vi "AuMT8852B EDR Carrier Frequency and Modulation Configuration.vi"(5 "Settings":T1={"Low frequency selection"=enum."Use low frequency", "Medium frequency selection"=enum."Use medium frequency", "High frequency selection"=enum."Use high frequency", "Low TX frequency"=2402.0, "Low RX frequency"=2480.0, "Medium TX frequency"=2441.0, "Medium RX frequency"=2402.0, "High TX frequency"=2480.0, "High RX frequency"=2402.0, "Number of blocks"=200, "Initial frequency error lower limit"=-75000.0, "Initial frequency error upper limit"=75000.0, "2DHx test packet"=enum."Longest", "3DHx test packet"=enum."Longest", "Hop selection"=enum."Test with hopping off", "Test control"=enum."Loopback", "Hop mode"=enum."Defined", "Frequency error lower limit"=-10000.0, "Frequency error upper limit"=10000.0, "Block frequency error lower limit"=-75000.0, "Block frequency error upper limit"=75000.0, "2Mbs RMS DEVM limit"=0.2, "3Mbs RMS DEVM limit"=0.13, "2Mbs peak DEVM limit"=0.35000000000000014, "3Mbs peak DEVM limit"=0.25, "2Mbs 99% packets DEVM limit"=0.3, "3Mbs 99% packets DEVM limit"=0.2} {"3Mbs 99% packets DEVM limit" min=0.0 max=1.0 step=0.01 format="%.2f"; "2Mbs 99% packets DEVM limit" min=0.0 max=1.0 step=0.01 format="%.2f"; "3Mbs peak DEVM limit" min=0.0 max=1.0 step=0.01 format="%.2f"; "2Mbs peak DEVM limit" min=0.0 max=1.0 step=0.01 format="%.2f"; "3Mbs RMS DEVM limit" min=0.0 max=1.0 step=0.01 format="%.2f"; "2Mbs RMS DEVM limit" min=0.0 max=1.0 step=0.01 format="%.2f"; "Block frequency error upper limit" min=-100000.0 max=100000.0 step=1000.0 format="%#.0f"; "Block frequency error lower limit" min=-100000.0 max=100000.0 step=1000.0 format="%#.2f"; "Frequency error upper limit" min=-100000.0 max=100000.0 step=1000.0 format="%#.0f"; "Frequency error lower limit" min=-100000.0 max=100000.0 step=1000.0 format="%#.0f"; "Initial frequency error upper limit" min=-100000.0 max=100000.0 step=1000.0 format="%#.0f"; "Initial frequency error lower limit" min=-100000.0 max=100000.0 step=1000.0 format="%#.0f"}, 7 "Set/Get (Set)":enum16{"Set", "Get"}(ring), 8 "error in (no error)":errorcluster, 10 "Script (3)":i32=3, 11 "VISA session":refnum<visa-resource-name>) -> (0 "error out":errorcluster, 2 "error code":i32, 3 "VISA session out":refnum<visa-resource-name>, 4 "Settings out":T1={"Low frequency selection"=enum."Use low frequency", "Medium frequency selection"=enum."Use medium frequency", "High frequency selection"=enum."Use high frequency", "Low TX frequency"=2402.0, "Low RX frequency"=2480.0, "Medium TX frequency"=2441.0, "Medium RX frequency"=2402.0, "High TX frequency"=2480.0, "High RX frequency"=2402.0, "Number of blocks"=200, "Initial frequency error lower limit"=-75000.0, "Initial frequency error upper limit"=75000.0, "2DHx test packet"=enum."Longest", "3DHx test packet"=enum."Longest", "Hop selection"=enum."Test with hopping off", "Test control"=enum."Loopback", "Hop mode"=enum."Defined", "Frequency error lower limit"=-10000.0, "Frequency error upper limit"=10000.0, "Block frequency error lower limit"=-75000.0, "Block frequency error upper limit"=75000.0, "2Mbs RMS DEVM limit"=0.2, "3Mbs RMS DEVM limit"=0.13, "2Mbs peak DEVM limit"=0.35000000000000014, "3Mbs peak DEVM limit"=0.25, "2Mbs 99% packets DEVM limit"=0.3, "3Mbs 99% packets DEVM limit"=0.2} {"3Mbs 99% packets DEVM limit" format="%.2f"; "2Mbs 99% packets DEVM limit" format="%.2f"; "3Mbs peak DEVM limit" format="%.2f"; "2Mbs peak DEVM limit" format="%.2f"; "3Mbs RMS DEVM limit" format="%.2f"; "2Mbs RMS DEVM limit" format="%.2f"; "Block frequency error upper limit" format="%#.2f"; "Block frequency error lower limit" format="%#.2f"; "Frequency error upper limit" format="%#.2f"; "Frequency error lower limit" format="%#.2f"; "Initial frequency error upper limit" format="%#.0f"; "Initial frequency error lower limit" format="%#.2f"})   [LabVIEW 2017]
doc: "Anritsu MT8852B Bluetooth Tester\n\nConfigures the instrument for the EDR Carrier Frequency Stability and Modulation test.\n\nINPUTS\nSet/Get - whether the values are being sent to or retrieved from the instrument.\nScript - which of the stored scripts (1-10) will be queried or configured. Scripts 1 and 2 are read-only.\nSettings - parameters of the test to be written.\n\nOUTPUTS\nSettings out - current parameters of the test."
uses:
  <instrlib>/aumt8852B/General/Utilities/MT8850 Test Parameters.ctl
  <instrlib>/aumt8852B/General/Utilities/MT8850 Frequency Units.ctl
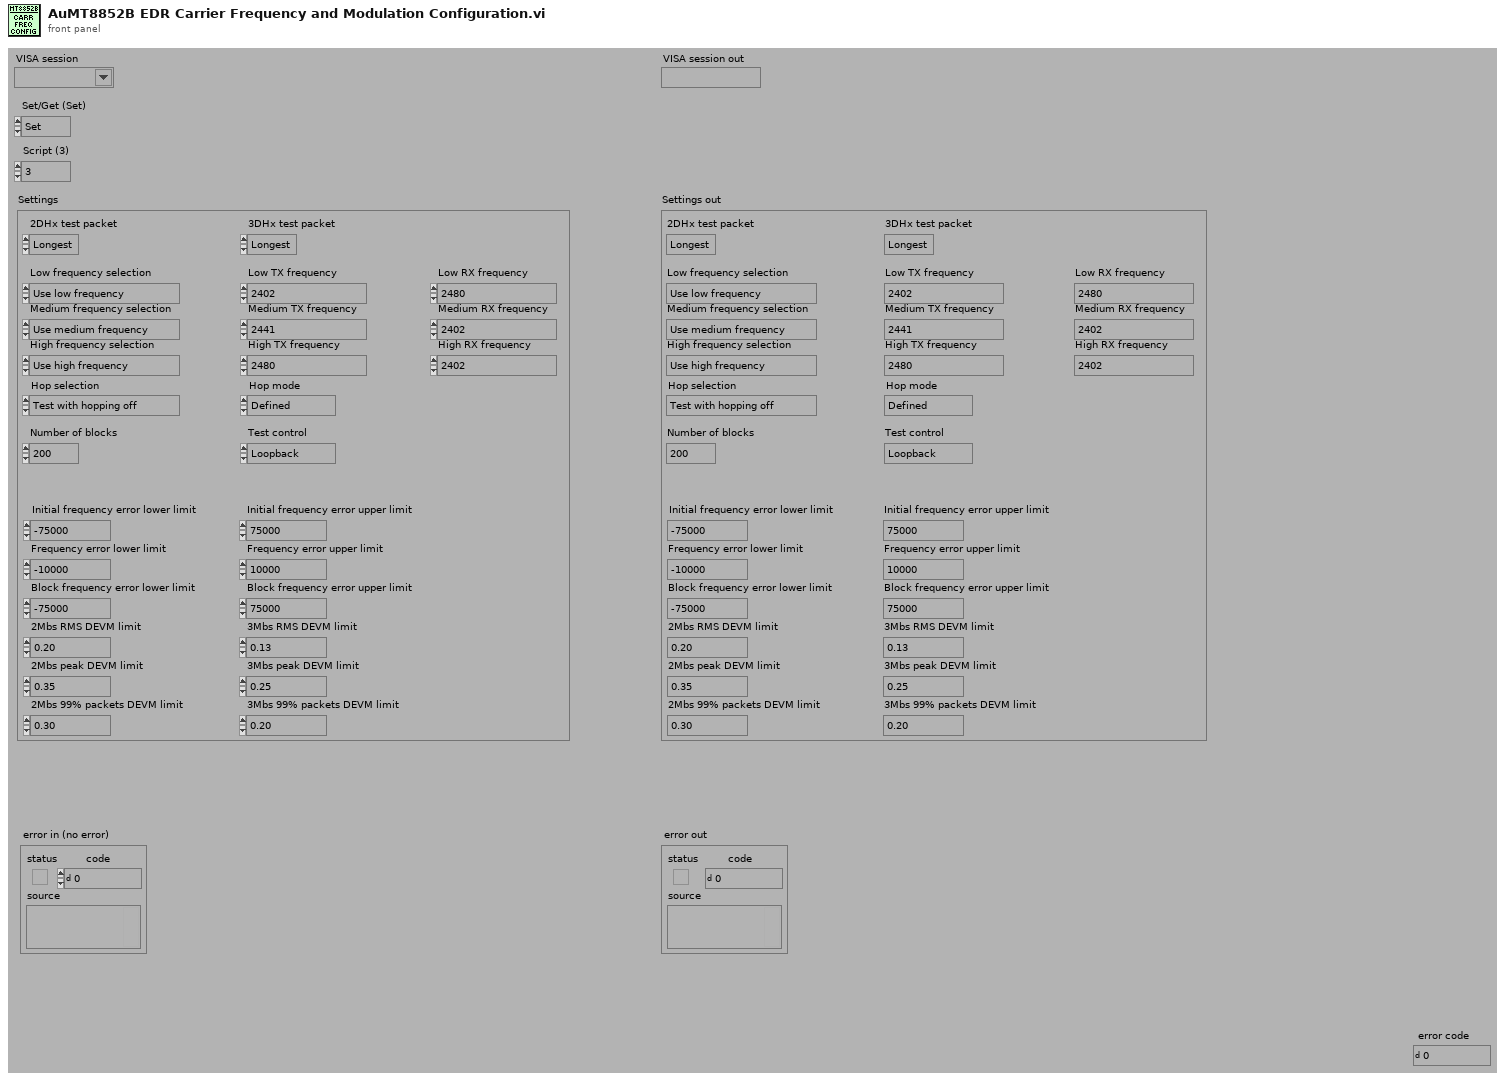
[diagram p1: front panel]
types:
  T1 = cluster{"Low frequency selection":enum16{"Don't use low frequency", "Use low frequency"}, "Medium frequency selection":enum16{"Don't use medium frequency", "Use medium frequency"}, "High frequency selection":enum16{"Don't use high frequency", "Use high frequency"}, "Low TX frequency":dbl, "Low RX frequency":dbl, "Medium TX frequency":dbl, "Medium RX frequency":dbl, "High TX frequency":dbl, "High RX frequency":dbl, "Number of blocks":i32, "Initial frequency error lower limit":dbl, "Initial frequency error upper limit":dbl, "2DHx test packet":enum16{"OFF", "Longest", "2-DH1", "2-DH3", "2-DH5"}, "3DHx test packet":enum16{"OFF", "Longest", "3-DH1", "3-DH3", "3-DH5"}, "Hop selection":enum16{"Test with hopping on", "Test with hopping off", "Test with hopping off and on"}, "Test control":enum16{"Loopback", "TX test"}, "Hop mode":enum16{"All", "Any", "Defined"}, "Frequency error lower limit":dbl, "Frequency error upper limit":dbl, "Block frequency error lower limit":dbl, "Block frequency error upper limit":dbl, "2Mbs RMS DEVM limit":dbl, "3Mbs RMS DEVM limit":dbl, "2Mbs peak DEVM limit":dbl, "3Mbs peak DEVM limit":dbl, "2Mbs 99% packets DEVM limit":dbl, "3Mbs 99% packets DEVM limit":dbl}
  T2 = typedef "MT8850 Frequency Units.ctl" = enum16{"Channel", "Hz", "kHz", "MHz", "GHz"}
  T3 = typedef "MT8850 Test Parameters.ctl" = enum16{"Use low frequency", "Use medium frequency", "Use high frequency", "Low TX frequency", "Low RX frquency", "Medium TX frequency", "Medium RX frequency", "High TX frequency", "High RX frequency", "Number of packets", "Average high limit", "Average low limit", "Peak power limit", "Max power step limit", "Min power step limit", "f1 average minimum", "f1 average maximum", "f2 maximum", "f1/f2 average maximum", "Hop selection", "Use DH1 packets", "Use DH3 packets", "Use DH5 packets", "1 slot packet drift limit", "3 slot packet drift limit", "5 slot packet drift limit", "Drift rate limit", "TX power level", "Frequency offset", "Symbol timing", "Modulation index", "BER limit", "FER limit", "Use averaging high limit", "Use averaging low limit", "Use peak power limit", "Packet type", "Test control", "Use max power step limit", "Use min power step limit", "Number of cycles", "Use f1 average maximum", "Use f1 average minimum", "Use f2 maximum", "Use f1/f2 average maximum", "Hop mode", "Maximum negative limit", "Maximum positive limit", "Use maximum negative limit", "Use maximum positive limit", "Use 1 slot packet drift limit", "Use 3 slot packet drift limit", "Use 5 slot packet drift limit", "Use drift rate limit", "Use BER limit", "Use FER limit", "Use dirty parameter table", "Use null packet drift limit", "Null packet drift limit", "Minimum power", "Power delay", "Packet count", "Payload toggle", "Output power level", "2DHX packet type", "3DHX packet type", "Number of blocks", "TX and RX low frequency", "TX and RX medium frequency", "TX and RX high frequency", "TX frequency", "RX frequency", "Threshold bit count", "Total test bit count", "Number of bits", "PDPSK to PGFSK lower limit", "PDPSK to PGFSK upper limit", "Initial frequency error upper limit", "Initial frequency error lower limit", "Frequency error upper limit", "Frequency error lower limit", "Block frequency error upper limit", "Block frequency error lower limit", "2Mbs RMS DEVM limit", "3Mbs RMS DEVM limit", "2Mbs Peak DEVM limit", "3Mbs Peak DEVM limit", "2Mbs 99% packets DEVM limit", "3Mbs 99% packets DEVM limit", "Percentage of no error packets limit", "Threshold error limit", "Total test error limit"}
  T4 = enum16{"Output power", "Power control", "Modulation characteristics", "Initial carrier", "Carrier drift", "Single slot sensitivity", "Multiple slot sensitivity", "Maximum input power", "EDR Relative transmit power", "EDR Carrier frequency and stability", "EDR Differential phase encoding", "EDR Sensitivity", "EDR BER floor sensitivity", "EDR Maximum input power"}
  T5 = enum16{"Simulate", "Range check", "Cache", "Query instrument status"}
  T6 = enum16{"Test with hopping on", "Test with hopping off", "Test with hopping off and on"}
  T7 = enum16{"OFF", "Longest", "3-DH1", "3-DH3", "3-DH5"}
  T8 = enum16{"OFF", "Longest", "2-DH1", "2-DH3", "2-DH5"}
  T9 = enum16{"Don't use high frequency", "Use high frequency"}
  T10 = enum16{"Don't use medium frequency", "Use medium frequency"}
  T11 = enum16{"Don't use low frequency", "Use low frequency"}
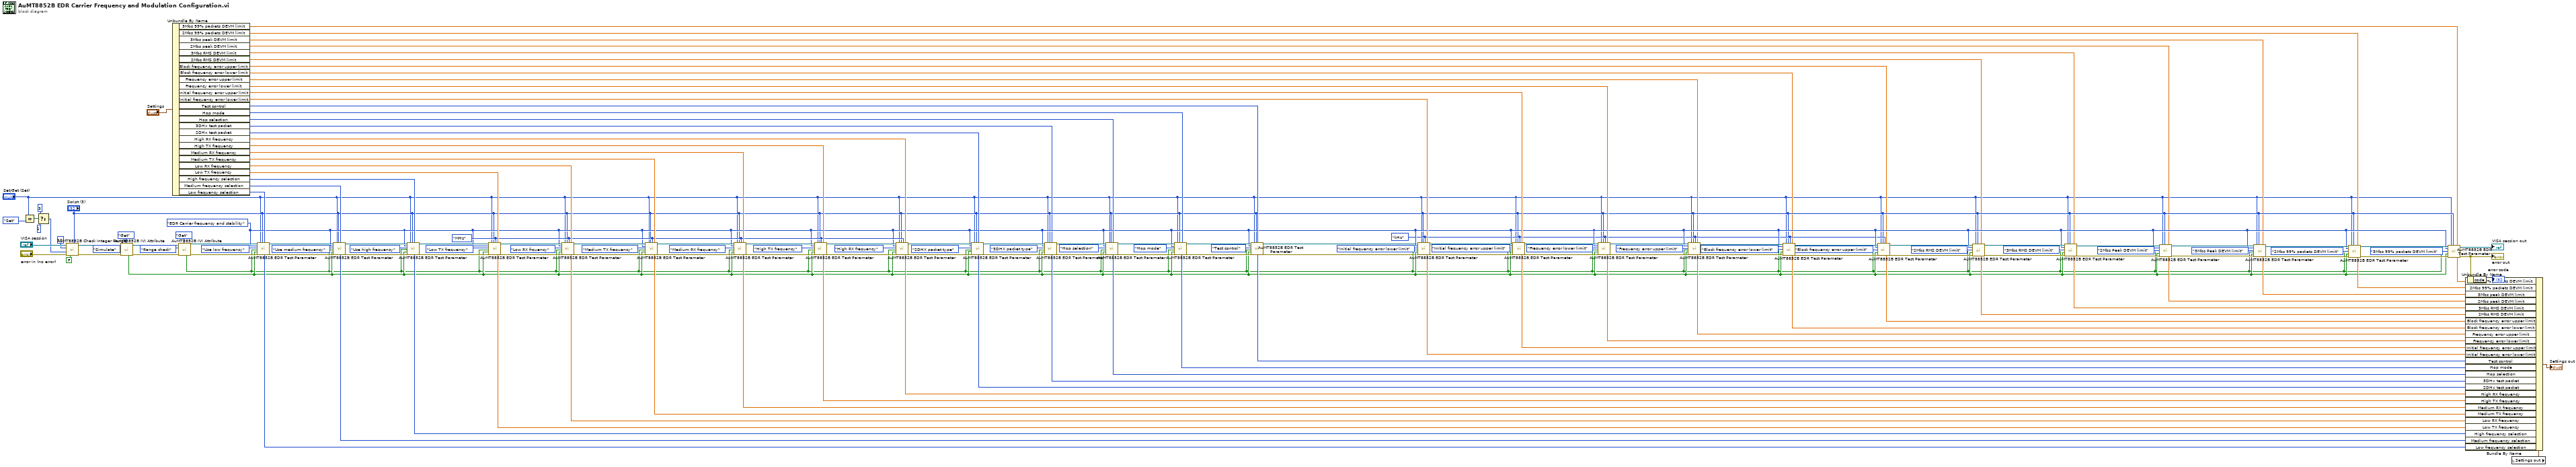
[diagram p0: block diagram]
diagram:
  w17 = MT8850_Frequency_Units."kHz" ("Frequency units (MHz)")
  w18 = T4."EDR Carrier frequency and stability" ("Test (Output power)")
  w85 = MT8850_Frequency_Units."MHz" ("Frequency units (MHz)")
  n1 = Equal?(x="Set/Get (Set)", y=enum16{"Set", "Get"}."Set") -> (x = y?=w157:bool)
  n2 = Select(t=3, s=w157, f=1) -> (s? t:f=w153:i32)
  n3 = call <instrlib>:"AuMT8852B Check Integer Range.vi"("Value (0)"="Script (3)", "Check IVI flag first? (T)"=FALSE, "error in (no error)"="error in (no error)", "Lower limit (-1)"=w153, "Upper limit (1)"=10, "VISA session"="VISA session") -> ("error out"=w151:errorcluster, "VISA session out"=w152:refnum<visa-resource-name>)  [unwired: 4 in]
  n4 = call <instrlib>:"AuMT8852B IVI Attribute.vi"("Set/Get (Set)"=enum16{"Set", "Get"}."Get", "error in (no error)"=w151, "Flag (Simulate)"=T5."Simulate", "VISA session"=w152) -> ("error out"=w125:errorcluster, "VISA session out"=w126:refnum<visa-resource-name>, "Value out"=w6:bool)  [unwired: 5 in]
  n5 = Unbundle By Name("Settings") -> ("3Mbs 99% packets DEVM limit"=w7:dbl, "2Mbs 99% packets DEVM limit"=w8:dbl, "3Mbs peak DEVM limit"=w9:dbl, "2Mbs peak DEVM limit"=w10:dbl, "3Mbs RMS DEVM limit"=w11:dbl, "2Mbs RMS DEVM limit"=w12:dbl, "Block frequency error upper limit"=w13:dbl, "Block frequency error lower limit"=w14:dbl, "Frequency error upper limit"=w15:dbl, "Frequency error lower limit"=w61:dbl, "Initial frequency error upper limit"=w62:dbl, "Initial frequency error lower limit"=w19:dbl, "Test control"=w73:enum16{"Loopback", "TX test"}, "Hop mode"=w74:enum16{"All", "Any", "Defined"}, "Hop selection"=w78:T6, "3DHx test packet"=w4:T7, "2DHx test packet"=w99:T8, "High RX frequency"=w112:dbl, "High TX frequency"=w113:dbl, "Medium RX frequency"=w100:dbl, "Medium TX frequency"=w114:dbl, "Low RX frequency"=w115:dbl, "Low TX frequency"=w116:dbl, "High frequency selection"=w117:T9, "Medium frequency selection"=w118:T10, "Low frequency selection"=w119:T11)
  n6 = call <instrlib>:"AuMT8852B IVI Attribute.vi"("Set/Get (Set)"=enum16{"Set", "Get"}."Get", "error in (no error)"=w125, "Flag (Simulate)"=T5."Range check", "VISA session"=w126) -> ("error out"=w123:errorcluster, "VISA session out"=w124:refnum<visa-resource-name>, "Value out"=w5:bool)  [unwired: 5 in]
  n7 = call <instrlib>:"AuMT8852B EDR Test Parameter.vi"("VISA session"=w124, "Test (Output power)"=w18, "Parameter (Use low frequency)"=MT8850_Test_Parameters."Use low frequency", "Range check? (F)"=w5, "Simulate? (F)"=w6, "error in (no error)"=w123, "Set/Get (Set)"="Set/Get (Set)", "Script (3)"="Script (3)", "Integer value (0)"=w119) -> ("Integer value out"=w104:i32, "VISA session out"=w91:refnum<visa-resource-name>, "error out"=w90:errorcluster)  [unwired: 7 in, 1 out]
  n8 = call <instrlib>:"AuMT8852B EDR Test Parameter.vi"("VISA session"=w91, "Test (Output power)"=w18, "Parameter (Use low frequency)"=MT8850_Test_Parameters."Use medium frequency", "Range check? (F)"=w5, "Simulate? (F)"=w6, "error in (no error)"=w90, "Set/Get (Set)"="Set/Get (Set)", "Script (3)"="Script (3)", "Integer value (0)"=w118) -> ("Integer value out"=w105:i32, "VISA session out"=w89:refnum<visa-resource-name>, "error out"=w88:errorcluster)  [unwired: 7 in, 1 out]
  n9 = call <instrlib>:"AuMT8852B EDR Test Parameter.vi"("VISA session"=w89, "Test (Output power)"=w18, "Parameter (Use low frequency)"=MT8850_Test_Parameters."Use high frequency", "Range check? (F)"=w5, "Simulate? (F)"=w6, "error in (no error)"=w88, "Set/Get (Set)"="Set/Get (Set)", "Script (3)"="Script (3)", "Integer value (0)"=w117) -> ("Integer value out"=w106:i32, "VISA session out"=w147:refnum<visa-resource-name>, "error out"=w146:errorcluster)  [unwired: 7 in, 1 out]
  n10 = call <instrlib>:"AuMT8852B EDR Test Parameter.vi"("VISA session"=w147, "Test (Output power)"=w18, "Parameter (Use low frequency)"=MT8850_Test_Parameters."Low TX frequency", "Range check? (F)"=w5, "Simulate? (F)"=w6, "error in (no error)"=w146, "Set/Get (Set)"="Set/Get (Set)", "Script (3)"="Script (3)", "Integer value (0)"=w85, "Float value (0)"=w116) -> ("Float value out"=w107:dbl, "VISA session out"=w145:refnum<visa-resource-name>, "error out"=w144:errorcluster)  [unwired: 6 in, 1 out]
  n11 = call <instrlib>:"AuMT8852B EDR Test Parameter.vi"("VISA session"=w145, "Test (Output power)"=w18, "Parameter (Use low frequency)"=MT8850_Test_Parameters."Low RX frquency", "Range check? (F)"=w5, "Simulate? (F)"=w6, "error in (no error)"=w144, "Set/Get (Set)"="Set/Get (Set)", "Script (3)"="Script (3)", "Integer value (0)"=w85, "Float value (0)"=w115) -> ("Float value out"=w108:dbl, "VISA session out"=w143:refnum<visa-resource-name>, "error out"=w142:errorcluster)  [unwired: 6 in, 1 out]
  n12 = call <instrlib>:"AuMT8852B EDR Test Parameter.vi"("VISA session"=w143, "Test (Output power)"=w18, "Parameter (Use low frequency)"=MT8850_Test_Parameters."Medium TX frequency", "Range check? (F)"=w5, "Simulate? (F)"=w6, "error in (no error)"=w142, "Set/Get (Set)"="Set/Get (Set)", "Script (3)"="Script (3)", "Integer value (0)"=w85, "Float value (0)"=w114) -> ("Float value out"=w109:dbl, "VISA session out"=w141:refnum<visa-resource-name>, "error out"=w140:errorcluster)  [unwired: 6 in, 1 out]
  n13 = call <instrlib>:"AuMT8852B EDR Test Parameter.vi"("VISA session"=w141, "Test (Output power)"=w18, "Parameter (Use low frequency)"=MT8850_Test_Parameters."Medium RX frequency", "Range check? (F)"=w5, "Simulate? (F)"=w6, "error in (no error)"=w140, "Set/Get (Set)"="Set/Get (Set)", "Script (3)"="Script (3)", "Integer value (0)"=w85, "Float value (0)"=w100) -> ("Float value out"=w102:dbl, "VISA session out"=w139:refnum<visa-resource-name>, "error out"=w138:errorcluster)  [unwired: 6 in, 1 out]
  n14 = call <instrlib>:"AuMT8852B EDR Test Parameter.vi"("VISA session"=w139, "Test (Output power)"=w18, "Parameter (Use low frequency)"=MT8850_Test_Parameters."High TX frequency", "Range check? (F)"=w5, "Simulate? (F)"=w6, "error in (no error)"=w138, "Set/Get (Set)"="Set/Get (Set)", "Script (3)"="Script (3)", "Integer value (0)"=w85, "Float value (0)"=w113) -> ("Float value out"=w110:dbl, "VISA session out"=w137:refnum<visa-resource-name>, "error out"=w136:errorcluster)  [unwired: 6 in, 1 out]
  n15 = call <instrlib>:"AuMT8852B EDR Test Parameter.vi"("VISA session"=w137, "Test (Output power)"=w18, "Parameter (Use low frequency)"=MT8850_Test_Parameters."High RX frequency", "Range check? (F)"=w5, "Simulate? (F)"=w6, "error in (no error)"=w136, "Set/Get (Set)"="Set/Get (Set)", "Script (3)"="Script (3)", "Integer value (0)"=w85, "Float value (0)"=w112) -> ("Float value out"=w111:dbl, "VISA session out"=w135:refnum<visa-resource-name>, "error out"=w134:errorcluster)  [unwired: 6 in, 1 out]
  n16 = call <instrlib>:"AuMT8852B EDR Test Parameter.vi"("VISA session"=w135, "Test (Output power)"=w18, "Parameter (Use low frequency)"=MT8850_Test_Parameters."2DHX packet type", "Range check? (F)"=w5, "Simulate? (F)"=w6, "error in (no error)"=w134, "Set/Get (Set)"="Set/Get (Set)", "Script (3)"="Script (3)", "Integer value (0)"=w99) -> ("Integer value out"=w101:i32, "VISA session out"=w96:refnum<visa-resource-name>, "error out"=w95:errorcluster)  [unwired: 7 in, 1 out]
  n17 = call <instrlib>:"AuMT8852B EDR Test Parameter.vi"("VISA session"=w96, "Test (Output power)"=w18, "Parameter (Use low frequency)"=MT8850_Test_Parameters."3DHX packet type", "Range check? (F)"=w5, "Simulate? (F)"=w6, "error in (no error)"=w95, "Set/Get (Set)"="Set/Get (Set)", "Script (3)"="Script (3)", "Integer value (0)"=w4) -> ("Integer value out"=w72:i32, "VISA session out"=w81:refnum<visa-resource-name>, "error out"=w82:errorcluster)  [unwired: 7 in, 1 out]
  n18 = call <instrlib>:"AuMT8852B EDR Test Parameter.vi"("VISA session"=w81, "Test (Output power)"=w18, "Parameter (Use low frequency)"=MT8850_Test_Parameters."Hop selection", "Range check? (F)"=w5, "Simulate? (F)"=w6, "error in (no error)"=w82, "Set/Get (Set)"="Set/Get (Set)", "Script (3)"="Script (3)", "Integer value (0)"=w78) -> ("Integer value out"=w71:i32, "VISA session out"=w80:refnum<visa-resource-name>, "error out"=w83:errorcluster)  [unwired: 7 in, 1 out]
  n19 = call <instrlib>:"AuMT8852B EDR Test Parameter.vi"("VISA session"=w80, "Test (Output power)"=w18, "Parameter (Use low frequency)"=MT8850_Test_Parameters."Hop mode", "Range check? (F)"=w5, "Simulate? (F)"=w6, "error in (no error)"=w83, "Set/Get (Set)"="Set/Get (Set)", "Script (3)"="Script (3)", "Integer value (0)"=w74) -> ("Integer value out"=w70:i32, "VISA session out"=w76:refnum<visa-resource-name>, "error out"=w77:errorcluster)  [unwired: 7 in, 1 out]
  n20 = call <instrlib>:"AuMT8852B EDR Test Parameter.vi"("VISA session"=w76, "Test (Output power)"=w18, "Parameter (Use low frequency)"=MT8850_Test_Parameters."Test control", "Range check? (F)"=w5, "Simulate? (F)"=w6, "error in (no error)"=w77, "Set/Get (Set)"="Set/Get (Set)", "Script (3)"="Script (3)", "Integer value (0)"=w73) -> ("Integer value out"=w69:i32, "VISA session out"=w2:refnum<visa-resource-name>, "error out"=w1:errorcluster)  [unwired: 7 in, 1 out]
  n21 = call <instrlib>:"AuMT8852B EDR Test Parameter.vi"("VISA session"=w2, "Test (Output power)"=w18, "Parameter (Use low frequency)"=MT8850_Test_Parameters."Initial frequency error lower limit", "Range check? (F)"=w5, "Simulate? (F)"=w6, "error in (no error)"=w1, "Set/Get (Set)"="Set/Get (Set)", "Script (3)"="Script (3)", "Integer value (0)"=w17, "Float value (0)"=w19) -> ("Float value out"=w20:dbl, "VISA session out"=w66:refnum<visa-resource-name>, "error out"=w68:errorcluster)  [unwired: 6 in, 1 out]
  n22 = call <instrlib>:"AuMT8852B EDR Test Parameter.vi"("VISA session"=w66, "Test (Output power)"=w18, "Parameter (Use low frequency)"=MT8850_Test_Parameters."Initial frequency error upper limit", "Range check? (F)"=w5, "Simulate? (F)"=w6, "error in (no error)"=w68, "Set/Get (Set)"="Set/Get (Set)", "Script (3)"="Script (3)", "Integer value (0)"=w17, "Float value (0)"=w62) -> ("Float value out"=w21:dbl, "VISA session out"=w65:refnum<visa-resource-name>, "error out"=w67:errorcluster)  [unwired: 6 in, 1 out]
  n23 = call <instrlib>:"AuMT8852B EDR Test Parameter.vi"("VISA session"=w65, "Test (Output power)"=w18, "Parameter (Use low frequency)"=MT8850_Test_Parameters."Frequency error lower limit", "Range check? (F)"=w5, "Simulate? (F)"=w6, "error in (no error)"=w67, "Set/Get (Set)"="Set/Get (Set)", "Script (3)"="Script (3)", "Integer value (0)"=w17, "Float value (0)"=w61) -> ("Float value out"=w22:dbl, "VISA session out"=w58:refnum<visa-resource-name>, "error out"=w59:errorcluster)  [unwired: 6 in, 1 out]
  n24 = call <instrlib>:"AuMT8852B EDR Test Parameter.vi"("VISA session"=w58, "Test (Output power)"=w18, "Parameter (Use low frequency)"=MT8850_Test_Parameters."Frequency error upper limit", "Range check? (F)"=w5, "Simulate? (F)"=w6, "error in (no error)"=w59, "Set/Get (Set)"="Set/Get (Set)", "Script (3)"="Script (3)", "Integer value (0)"=w17, "Float value (0)"=w15) -> ("Float value out"=w23:dbl, "VISA session out"=w55:refnum<visa-resource-name>, "error out"=w56:errorcluster)  [unwired: 6 in, 1 out]
  n25 = call <instrlib>:"AuMT8852B EDR Test Parameter.vi"("VISA session"=w55, "Test (Output power)"=w18, "Parameter (Use low frequency)"=MT8850_Test_Parameters."Block frequency error lower limit", "Range check? (F)"=w5, "Simulate? (F)"=w6, "error in (no error)"=w56, "Set/Get (Set)"="Set/Get (Set)", "Script (3)"="Script (3)", "Integer value (0)"=w17, "Float value (0)"=w14) -> ("Float value out"=w24:dbl, "VISA session out"=w49:refnum<visa-resource-name>, "error out"=w50:errorcluster)  [unwired: 6 in, 1 out]
  n26 = call <instrlib>:"AuMT8852B EDR Test Parameter.vi"("VISA session"=w49, "Test (Output power)"=w18, "Parameter (Use low frequency)"=MT8850_Test_Parameters."Block frequency error upper limit", "Range check? (F)"=w5, "Simulate? (F)"=w6, "error in (no error)"=w50, "Set/Get (Set)"="Set/Get (Set)", "Script (3)"="Script (3)", "Integer value (0)"=w17, "Float value (0)"=w13) -> ("Float value out"=w25:dbl, "VISA session out"=w51:refnum<visa-resource-name>, "error out"=w52:errorcluster)  [unwired: 6 in, 1 out]
  n27 = call <instrlib>:"AuMT8852B EDR Test Parameter.vi"("VISA session"=w51, "Test (Output power)"=w18, "Parameter (Use low frequency)"=MT8850_Test_Parameters."2Mbs RMS DEVM limit", "Range check? (F)"=w5, "Simulate? (F)"=w6, "error in (no error)"=w52, "Set/Get (Set)"="Set/Get (Set)", "Script (3)"="Script (3)", "Float value (0)"=w12) -> ("Float value out"=w26:dbl, "VISA session out"=w37:refnum<visa-resource-name>, "error out"=w38:errorcluster)  [unwired: 7 in, 1 out]
  n28 = call <instrlib>:"AuMT8852B EDR Test Parameter.vi"("VISA session"=w37, "Test (Output power)"=w18, "Parameter (Use low frequency)"=MT8850_Test_Parameters."3Mbs RMS DEVM limit", "Range check? (F)"=w5, "Simulate? (F)"=w6, "error in (no error)"=w38, "Set/Get (Set)"="Set/Get (Set)", "Script (3)"="Script (3)", "Float value (0)"=w11) -> ("Float value out"=w27:dbl, "VISA session out"=w45:refnum<visa-resource-name>, "error out"=w46:errorcluster)  [unwired: 7 in, 1 out]
  n29 = call <instrlib>:"AuMT8852B EDR Test Parameter.vi"("VISA session"=w45, "Test (Output power)"=w18, "Parameter (Use low frequency)"=MT8850_Test_Parameters."2Mbs Peak DEVM limit", "Range check? (F)"=w5, "Simulate? (F)"=w6, "error in (no error)"=w46, "Set/Get (Set)"="Set/Get (Set)", "Script (3)"="Script (3)", "Float value (0)"=w10) -> ("Float value out"=w28:dbl, "VISA session out"=w39:refnum<visa-resource-name>, "error out"=w40:errorcluster)  [unwired: 7 in, 1 out]
  n30 = call <instrlib>:"AuMT8852B EDR Test Parameter.vi"("VISA session"=w39, "Test (Output power)"=w18, "Parameter (Use low frequency)"=MT8850_Test_Parameters."3Mbs Peak DEVM limit", "Range check? (F)"=w5, "Simulate? (F)"=w6, "error in (no error)"=w40, "Set/Get (Set)"="Set/Get (Set)", "Script (3)"="Script (3)", "Float value (0)"=w9) -> ("Float value out"=w29:dbl, "VISA session out"=w41:refnum<visa-resource-name>, "error out"=w42:errorcluster)  [unwired: 7 in, 1 out]
  n31 = call <instrlib>:"AuMT8852B EDR Test Parameter.vi"("VISA session"=w41, "Test (Output power)"=w18, "Parameter (Use low frequency)"=MT8850_Test_Parameters."2Mbs 99% packets DEVM limit", "Range check? (F)"=w5, "Simulate? (F)"=w6, "error in (no error)"=w42, "Set/Get (Set)"="Set/Get (Set)", "Script (3)"="Script (3)", "Float value (0)"=w8) -> ("Float value out"=w30:dbl, "VISA session out"=w34:refnum<visa-resource-name>, "error out"=w35:errorcluster)  [unwired: 7 in, 1 out]
  n32 = call <instrlib>:"AuMT8852B EDR Test Parameter.vi"("VISA session"=w34, "Test (Output power)"=w18, "Parameter (Use low frequency)"=MT8850_Test_Parameters."3Mbs 99% packets DEVM limit", "Range check? (F)"=w5, "Simulate? (F)"=w6, "error in (no error)"=w35, "Set/Get (Set)"="Set/Get (Set)", "Script (3)"="Script (3)", "Float value (0)"=w7) -> ("Float value out"=w31:dbl, "VISA session out"=→"VISA session out":refnum<visa-resource-name>, "error out"=w33:errorcluster)  [unwired: 7 in, 1 out]
  "error out" <- w33
  n33 = Unbundle By Name(w33) -> ("code"=→"error code":i32)
  n34 = local read "Settings out"() -> (w103:T1)
  n35 = Bundle By Name(cluster=w103, "3Mbs 99% packets DEVM limit"=w31, "2Mbs 99% packets DEVM limit"=w30, "3Mbs peak DEVM limit"=w29, "2Mbs peak DEVM limit"=w28, "3Mbs RMS DEVM limit"=w27, "2Mbs RMS DEVM limit"=w26, "Block frequency error upper limit"=w25, "Block frequency error lower limit"=w24, "Frequency error upper limit"=w23, "Frequency error lower limit"=w22, "Initial frequency error upper limit"=w21, "Initial frequency error lower limit"=w20, "Test control"=w69, "Hop mode"=w70, "Hop selection"=w71, "3DHx test packet"=w72, "2DHx test packet"=w101, "High RX frequency"=w111, "High TX frequency"=w110, "Medium RX frequency"=w102, "Medium TX frequency"=w109, "Low RX frequency"=w108, "Low TX frequency"=w107, "High frequency selection"=w106, "Medium frequency selection"=w105, "Low frequency selection"=w104) -> (→"Settings out":T1)
